vi "GetHint.vi"(8 "No Error":errorcluster, 11 "Hint Name":T1) -> (0 "error out":errorcluster, 2 "Found?":bool, 3 "Value":string)   [LabVIEW 2026, in "SDL3.lvlib" / "Hints.lvlib"]
doc: "<B>Summary</B>\nGet the value of a hint.\n\n<B>Remarks</B>\nHints will not be set if there is an existing override hint or environment variable that takes precedence. You can use <B>SDL_SetHintWithPriority()</B> to set the hint with override priority instead."
uses:
  Hints.lvlib
  HintName--combobox.ctl
  Stdinc/Strlen.vi
  Stdinc/Strlen.vi/c3f57b18-2899-4d18-8de7-ed42e0d99649.vi
  <vilib>/Utility/error.llb/Error Cluster From Error Code.vi
  LV-Utilities/LV-Utilities.lvlib
  Lib/SDL3.dll
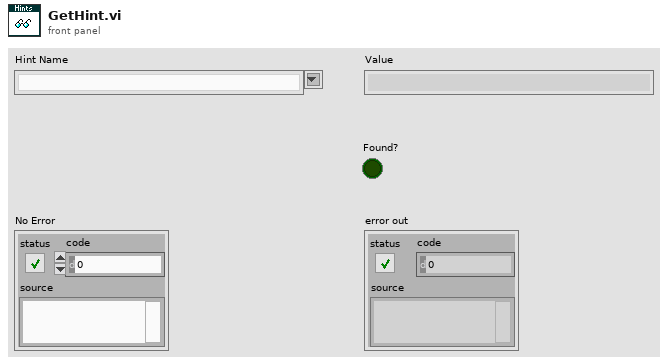
[diagram p1: front panel]
types:
  T1 = typedef "SDL3.lvlib/Hints.lvlib/HintName--combobox.ctl" = string
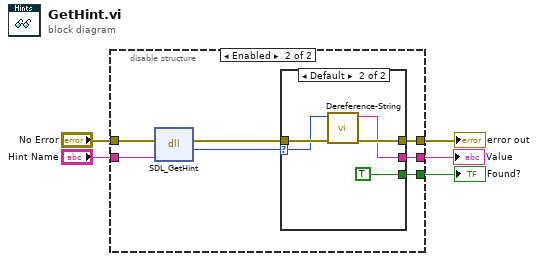
[diagram p0: block diagram]
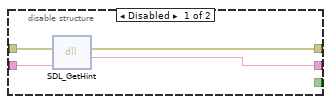
[diagram p2: hidden frame]
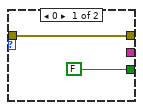
[diagram p3: hidden frame]
diagram:
  n1 = disable-structure shown="Enabled" {
    disable-tunnel: "No Error" -> [w9 w16]
    disable-tunnel: [w8 w14] -> w4
    disable-tunnel: "Hint Name" -> [w7 w15]
    disable-tunnel: [w6 w11] -> w2
    disable-tunnel: [_ w10] -> w1
    frame Disabled {
      n2 = dll-call lib="C:/Users/saukko/Dev/LV-SDL3/Sources/SDL3/Lib/SDL3.*" fn="SDL_GetHint"(error in=w9, "name"=w7) -> (error out=w8:errorcluster, "return type"=w6:string)  [unwired: 3 in, 1 out]
    }
    frame Enabled {
      n3 = dll-call lib="C:/Users/saukko/Dev/LV-SDL3/Sources/SDL3/Lib/SDL3.*" fn="SDL_GetHint"(error in=w16, "name"=w15) -> (error out=w13:errorcluster, "return type"=w12:i64)  [unwired: 3 in, 1 out]
      n4 = case shown="Default" w12 {
        selector: w12 -> [_ w20]
        tunnel: [w18 w21] -> w14
        tunnel: w13 -> [w18 w22]
        tunnel: [_ w19] -> w11
        tunnel: [FALSE TRUE] -> w10
        frame 0 {
        }
        frame Default {
          n5 = call "Dereference-String.vi"("No Error"=w22, "Str [const char *]"=w20) -> ("error out"=w21:errorcluster, "String"=w19:string)  [unwired: 8 in]
        }
      }
    }
  }
  "error out" <- w4
  "Value" <- w2
  "Found?" <- w1
